vi "Equal Within Tolerance.vi"(0 "Number In":dbl, 2 "Comparison Value":dbl, 8 "Tolerance":dbl=0.05) -> (15 "Equality":bool)   [LabVIEW 2012]
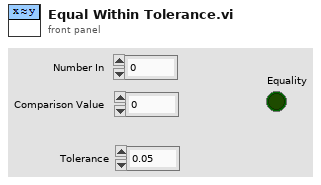
[diagram p1: front panel]
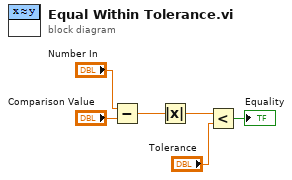
[diagram p0: block diagram]
diagram:
  n1 = Subtract(x="Number In", y="Comparison Value") -> (x-y=w3:dbl)
  n2 = Absolute Value(x=w3) -> (abs(x)=w2:dbl)
  n3 = Less?(x=w2, y="Tolerance") -> (x < y?=→"Equality":bool)
